vi "SetAvailable.vi"(6 "Param ID (Ring)":T1, 8 "error in (no error)":errorcluster, 11 "CameraSession in":refnum<class "CS250-CameraHardwareClass.lvclass">) -> (0 "error out":errorcluster, 3 "CameraSession out":refnum<class "CS250-CameraHardwareClass.lvclass">)   [LabVIEW 2013, in "CS250-CameraHardwareClass.lvclass"]
uses:
  CS250-CameraHardwareClass.lvclass
  SubVis/DLL Calls/PARAM_ID_TypDef.ctl
  CS250-CameraHardwareClass.lvclass/CS250-CameraHardwareClass.ctl
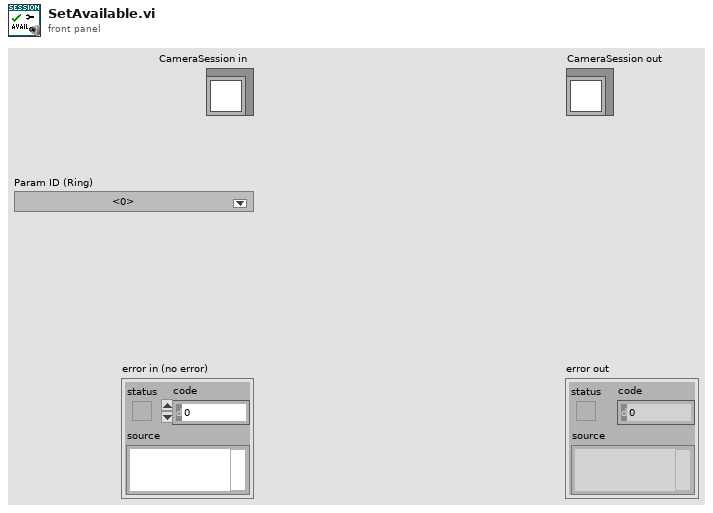
[diagram p1: front panel]
types:
  T1 = typedef "PARAM_ID_TypDef.ctl" = u32
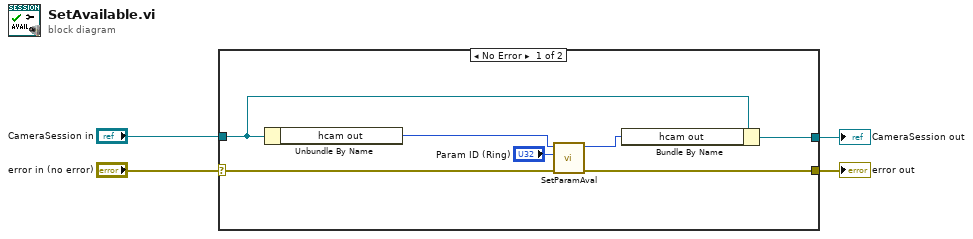
[diagram p0: block diagram]
diagram:
  n1 = case shown="No Error" "error in (no error)" {
    selector: "error in (no error)" -> [w10 w13]
    tunnel: [w9 w13] -> w3
    tunnel: [w6 w12] -> w1
    tunnel: "CameraSession in" -> [w8 w12]
    frame No Error {
      n2 = Unbundle By Name(w8) -> ("hcam out"=w11:i16)
      n3 = call "SetParamAval.vi"("error in (no error)"=w10, "Param ID (Ring)"="Param ID (Ring)", "hcam in"=w11) -> ("error out"=w9:errorcluster, "hcam out"=w7:i16)  [unwired: 6 in, 1 out]
      n4 = Bundle By Name(cluster=w8, "hcam out"=w7) -> (w6:refnum<class "CS250-CameraHardwareClass.lvclass">)
    }
    frame Error {
    }
  }
  "error out" <- w3
  "CameraSession out" <- w1
